vi "exercise3.vi"() -> ()   [LabVIEW 2025]
panel:
  in  "DC":dbl(knob) scale=0.0..10.0
  in  "V/div":dbl(knob) scale=0.0..10.0
  out "Waveform Graph":dbl[](graph)
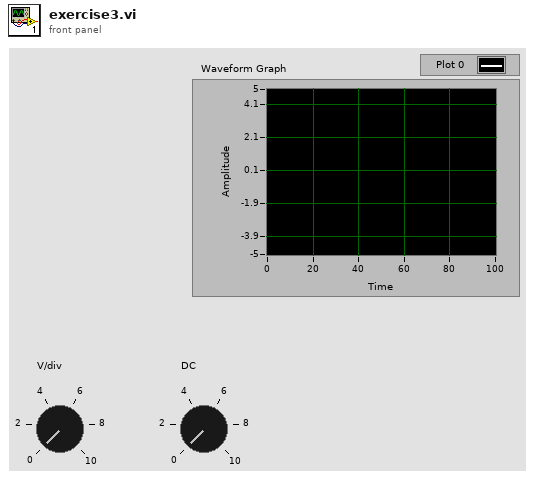
[diagram p1: front panel]
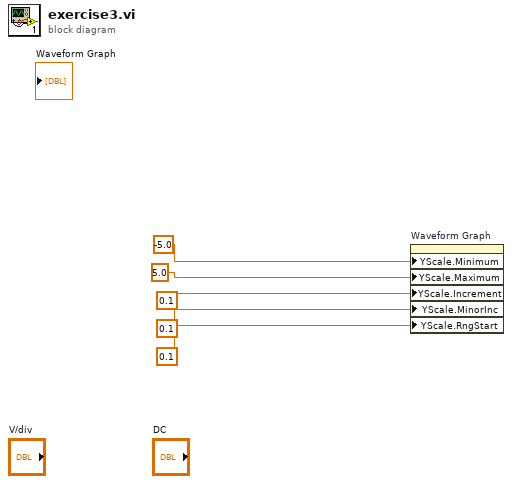
[diagram p0: block diagram]
diagram:
  n1 = property on="Waveform Graph" class="WFGraph (strict)"("YScale.Minimum"=-5.0, "YScale.Maximum"=5.0, "YScale.Increment"=0.1, "YScale.MinorInc"=0.1, "YScale.RngStart"=0.1) -> ()  [unwired: 2 in, 2 out]
